vi "Cycle Average and RMS 1 chan.vi"(6 "percent level settings":T2={"method"=enum."auto select", "histogram size"=256, "histogram method"=enum."mode", "reserved"=1.0} {"reserved" format="%0.2f"}, 7 "cycle number (1)":i32=1 min=1, 8 "error in (no error)":errorcluster, 9 "reference levels":T3={"high ref level"=90.0, "mid ref level"=50.0, "low ref level"=10.0, "ref units"=1} {"ref units" items=["absolute", "percent"]; "high ref level" format="%0.2f"; "low ref level" format="%0.2f"; "mid ref level" format="%0.2f"}, 11 "signal in":waveform(dbl)={"t0"=timestamp(0 s since 1904-01-01), "dt"=0.0, "Y"=[]}) -> (0 "error out":errorcluster, 2 "cycle RMS":dbl format="%.2g", 3 "cycle average":dbl format="%.2p", 4 "measurement info":T1 {"ref levels"."ref units" items=["absolute", "relative"]; "ref levels"."high ref level" format="%.2p"; "ref levels"."low ref level" format="%.2p"; "ref levels"."mid ref level" format="%.2p"; "end time" format="%.2p"; "start time" format="%.2p"})   [LabVIEW 2020, in "NI_MAPro.lvlib"]
doc: "Returns the average and RMS levels of a selected cycle of a periodic waveform or an array of periodic waveforms. Wire data to the <B>signal in</B> input to determine the polymorphic instance to use or manually select the instance."
uses:
  NI_MAPro.lvlib
  NI_MABase.lvlib
  <resource>/lvanlys.dll
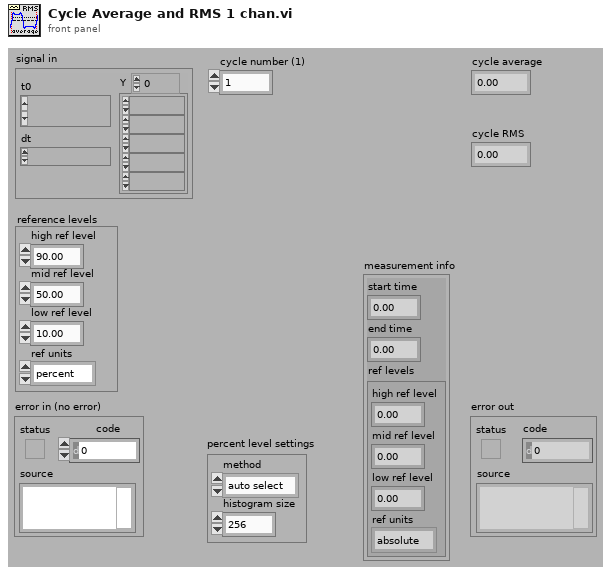
[diagram p1: front panel]
types:
  T1 = cluster{"start time":dbl, "end time":dbl, "ref levels":cluster{"high ref level":dbl, "mid ref level":dbl, "low ref level":dbl, "ref units":u16}}
  T2 = cluster{"method":enum32{"histogram", "peak", "auto select"}, "histogram size":i32, "histogram method":enum16{"mode"}, "reserved":dbl}
  T3 = cluster{"high ref level":dbl, "mid ref level":dbl, "low ref level":dbl, "ref units":u16}
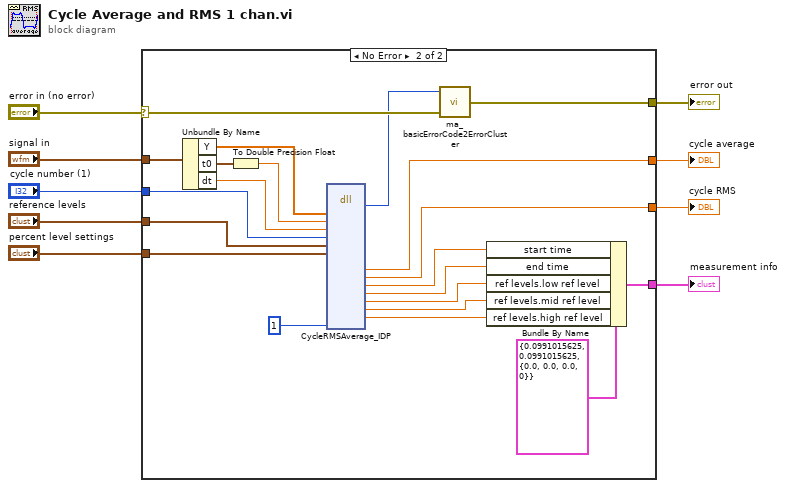
[diagram p0: block diagram]
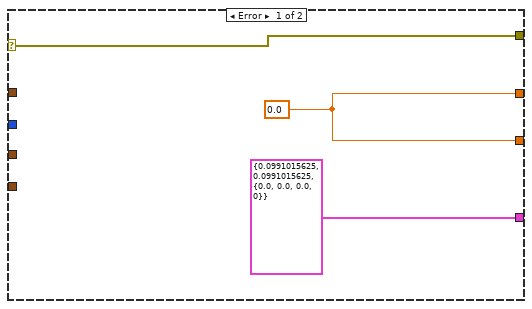
[diagram p2: hidden frame]
diagram:
  n1 = case shown="No Error" "error in (no error)" {
    selector: "error in (no error)" -> [w12 w32]
    tunnel: "reference levels" -> [_ w26]
    tunnel: "percent level settings" -> [_ w27]
    tunnel: "cycle number (1)" -> [_ w28]
    tunnel: "signal in" -> [_ w33]
    tunnel: [w12 w31] -> w4
    tunnel: [w11 w29] -> w3
    tunnel: [w11 w30] -> w2
    tunnel: [T1 {"start time"=0.0991015625, "end time"=0.0991015625, "ref levels"={"high ref level"=0.0, "mid ref level"=0.0, "low ref level"=0.0, "ref units"=0}} ("measurement info") w25] -> w1
    frame Error {
      w11 = 0.0 ("result")
    }
    frame No Error {
      n2 = Unbundle By Name(w33) -> ("Y"=w24:dbl[], "t0"=w23:timestamp, "dt"=w21:dbl)
      n3 = To Double Precision Float(number=w23) -> (double precision float=w22:dbl)
      n4 = dll-call lib="C:/Program Files (x86)/National Instruments/LabVIEW 2020/resource/lvanlys.*" fn="CycleRMSAverage_IDP" ("lvanlys_debug.dll:CycleRMSAverage")("xH"=w24, "Xo"=w22, "dx"=w21, "cycleNum"=w28, "refLevel"=w26, "percentLevel"=w27, "newAlgorithm"=1) -> ("return type"=w18:i32, "cycleAvg"=w29:dbl, "cycleRMS"=w30:dbl, "startingTime"=w20:dbl, "endingTime"=w17:dbl, "lowRefLevel"=w16:dbl, "midRefLevel"=w14:dbl, "highRefLevel"=w15:dbl)  [unwired: 10 in, 11 out]
      n5 = call "ma_basicErrorCode2ErrorCluster.vi"("error in (no error)"=w32, "Error Code"=w18) -> ("error out"=w31:errorcluster)  [unwired: 1 in]
      n6 = Bundle By Name(cluster=T1 {"start time"=0.0991015625, "end time"=0.0991015625, "ref levels"={"high ref level"=0.0, "mid ref level"=0.0, "low ref level"=0.0, "ref units"=0}} ("measurement info"), "start time"=w20, "end time"=w17, "ref levels.low ref level"=w16, "ref levels.mid ref level"=w14, "ref levels.high ref level"=w15) -> (w25:T1)
    }
  }
  "cycle average" <- w3
  "cycle RMS" <- w2
  "error out" <- w4
  "measurement info" <- w1
